vi "ModeDrivebase.vi"(0 "Master State In":T1(ring)) -> (1 "Drive Mode Change":bool, 2 "Drive Mode":enum16{"Driver Control", "Lock Heading"}(ring), 3 "Locked Heading (deg)":dbl)   [LabVIEW 2020]
doc: "This VI manages the robot drivebase mode. The default mode is driver control in which the swerve drive accepts all drive inputs and seemlessly combines them with autonomous heading corrections. Two auto targeting modes are also implimented."
uses:
  <vilib>/Rock Robotics/WPI/DriverStation/WPI_DriverStationAllianceInfo.ctl
  74109b1a-375b-4193-a712-f625c004fbb2.vi
  654a9305-fb99-4107-9368-618fc6918f82.vi
  fc0623c4-a7ba-4d2c-8dc2-a77ada9ce4c8.vi
  434b5739-c420-4379-a725-382a96265523.vi
  GlobalDriverStationCommands.vi
  GlobalPoseAndTargeting.vi
  GlobalDriverStationData.vi
  GlobalDrivebase.vi
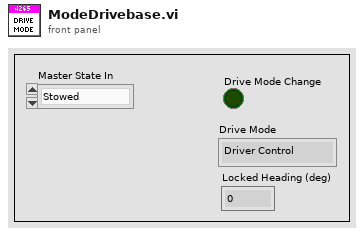
[diagram p1: front panel]
types:
  T1 = enum16{"Stowed", "Balancing", "Scoring", "Hoppering", "Ground", "Shelf"}
  T2 = enum16{"AutoTargeting", "Driver Control", "Lock Heading"}
  T3 = typedef "WPI_DriverStationAllianceInfo.ctl" = enum16{"Red", "Blue", "Invalid"}
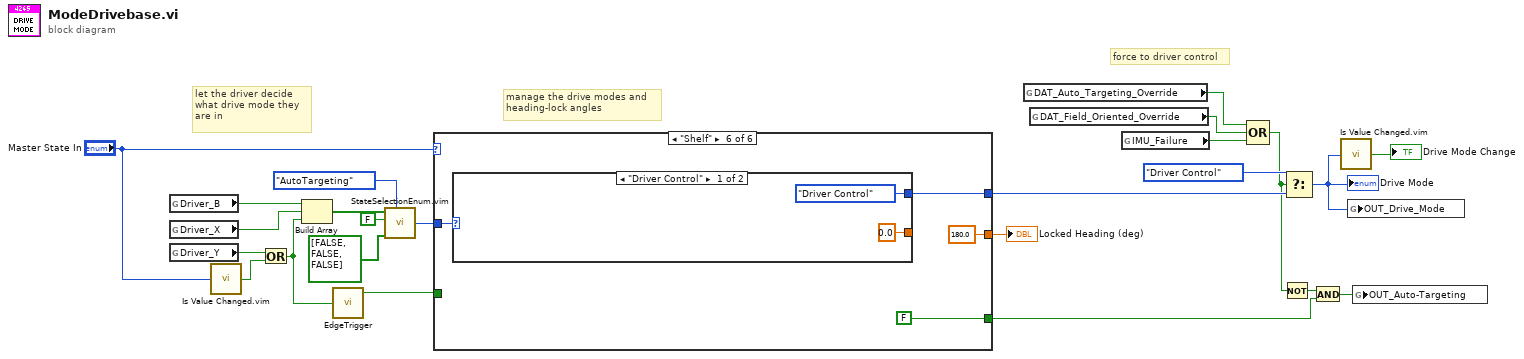
[diagram p0: block diagram]
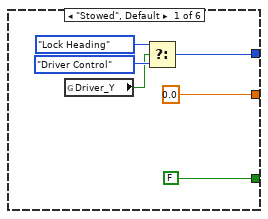
[diagram p2: hidden frame]
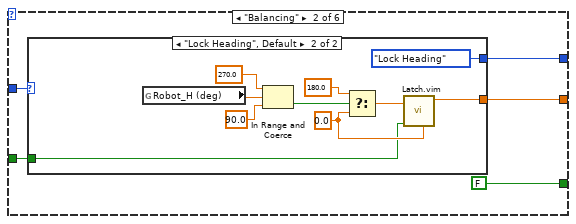
[diagram p3: hidden frame]
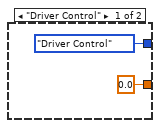
[diagram p4: hidden frame]
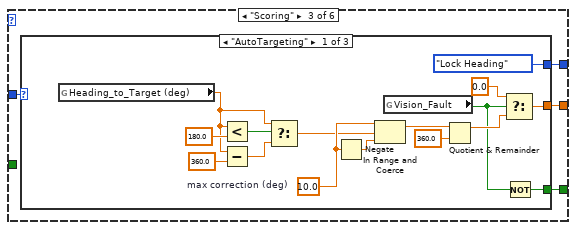
[diagram p5: hidden frame]
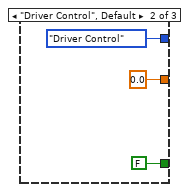
[diagram p6: hidden frame]
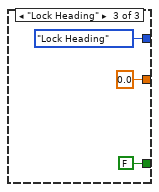
[diagram p7: hidden frame]
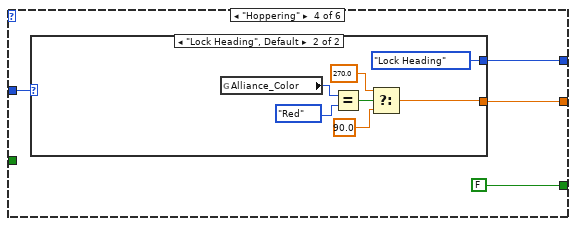
[diagram p8: hidden frame]
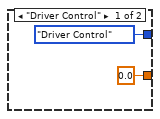
[diagram p9: hidden frame]
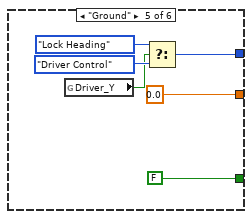
[diagram p10: hidden frame]
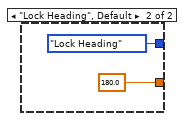
[diagram p11: hidden frame]
diagram:
  # "manage the drive modes and\nheading-lock angles"
  # "let the driver decide\nwhat drive mode they\nare in"
  # "force to driver control"
  n1 = global read "GlobalDriverStationCommands.vi" "Driver_B"() -> (w7:bool)
  n2 = global read "GlobalDriverStationCommands.vi" "Driver_X"() -> (w24:bool)
  n3 = global read "GlobalDriverStationCommands.vi" "Driver_Y"() -> (w23:bool)
  n4 = call "Is Value Changed.vim"("value"="Master State In") -> ("changed or first call?"=w13:bool)
  n5 = Or(x=w23, y=w13) -> (x .or. y?=w6:bool)
  n6 = Build Array(w7, w24, w6) -> (w22:bool[])
  n7 = call "EdgeTrigger.vi"("Input Signal"=w6) -> ("Rising Edge Trigger"=w5:bool)  [unwired: 2 out]
  n8 = call "StateSelectionEnum.vim"("Enum Def"=T2."AutoTargeting" ("Drive Mode"), "Disallowed States"=bool[] [FALSE, FALSE, FALSE], "Enable Edge Trigger"=FALSE, "State Triggers"=w22) -> ("Selected State"=w16:T2)  [unwired: 1 in, 1 out]
  n9 = case shown="\"Shelf\"" "Master State In" {
    tunnel: w16 -> [_ w33 w51 w75 _ w95]
    tunnel: [w27 w35 w50 w77 w87 w96] -> w15
    tunnel: [0.0 w34 w49 w76 0.0 180.0 ("f")] -> w14
    tunnel: w5 -> [_ w32 _ _ _ _]
    tunnel: [FALSE FALSE w48 FALSE FALSE FALSE] -> w2
    frame "Stowed", Default {
      n10 = global read "GlobalDriverStationCommands.vi" "Driver_Y"() -> (w25:bool)
      n11 = Select(t=enum16{"Driver Control", "Lock Heading"}."Lock Heading" ("Drive Mode"), s=w25, f=enum16{"Driver Control", "Lock Heading"}."Driver Control" ("Drive Mode")) -> (s? t:f=w27:enum16{"Driver Control", "Lock Heading"})
    }
    frame "Balancing" {
      n12 = case shown="\"Lock Heading\", Default" w33 {
        tunnel: [enum16{"Driver Control", "Lock Heading"}."Driver Control" ("Drive Mode") enum16{"Driver Control", "Lock Heading"}."Lock Heading" ("Drive Mode")] -> w35
        tunnel: [0.0 w40] -> w34
        tunnel: w32 -> [_ w38]
        frame "Driver Control" {
        }
        frame "Lock Heading", Default {
          w39 = 0.0 ("f")
          n13 = global read "GlobalPoseAndTargeting.vi" "Robot_H (deg)"() -> (w45:dbl)
          n14 = In Range and Coerce(upper limit=270.0, x=w45, lower limit=90.0) -> (In Range?=w46:bool)  [unwired: 1 out]
          n15 = Select(t=180.0, s=w46, f=w39) -> (s? t:f=w41:dbl)
          n16 = call "Latch.vim"("Default Value"=w39, "Latch Signal"=w38, "Latch Value"=w41) -> ("Latched"=w40:dbl)  [unwired: 8 in]
        }
      }
    }
    frame "Scoring" {
      n17 = case shown="\"AutoTargeting\"" w51 {
        tunnel: [enum16{"Driver Control", "Lock Heading"}."Lock Heading" ("Drive Mode") enum16{"Driver Control", "Lock Heading"}."Driver Control" ("Drive Mode") enum16{"Driver Control", "Lock Heading"}."Lock Heading" ("Drive Mode")] -> w50
        tunnel: [w56 0.0 0.0] -> w49
        tunnel: [w53 FALSE FALSE] -> w48
        frame "AutoTargeting" {
          w65 = 10.0  # max correction (deg)
          n18 = global read "GlobalPoseAndTargeting.vi" "Heading_to_Target (deg)"() -> (w59:dbl)
          n19 = Less?(x=w59, y=180.0) -> (x < y?=w62:bool)
          n20 = Subtract(x=w59, y=360.0) -> (x-y=w58:dbl)
          n21 = Select(t=w59, s=w62, f=w58) -> (s? t:f=w57:dbl)
          n22 = Negate(x=w65) -> (-x=w64:dbl)
          n23 = In Range and Coerce(upper limit=w65, x=w57, lower limit=w64) -> (coerced(x)=w67:dbl)  [unwired: 1 out]
          n24 = global read "GlobalPoseAndTargeting.vi" "Vision_Fault"() -> (w52:bool)
          n25 = Quotient & Remainder(x=w67, y=360.0) -> (x-y*floor(x/y)=w55:dbl)  [unwired: 1 out]
          n26 = Select(t=0.0, s=w52, f=w55) -> (s? t:f=w56:dbl)
          n27 = Not(x=w52) -> (.not. x?=w53:bool)
        }
        frame "Driver Control", Default {
        }
        frame "Lock Heading" {
        }
      }
    }
    frame "Hoppering" {
      n28 = case shown="\"Lock Heading\", Default" w75 {
        tunnel: [enum16{"Driver Control", "Lock Heading"}."Driver Control" ("Drive Mode") enum16{"Driver Control", "Lock Heading"}."Lock Heading" ("Drive Mode")] -> w77
        tunnel: [0.0 w80] -> w76
        frame "Driver Control" {
        }
        frame "Lock Heading", Default {
          n29 = global read "GlobalDriverStationData.vi" "Alliance_Color"() -> (w85:T3)
          n30 = Equal?(x=w85, y=WPI_DriverStationAllianceInfo."Red") -> (x = y?=w83:bool)
          n31 = Select(t=270.0, s=w83, f=90.0) -> (s? t:f=w80:dbl)
        }
      }
    }
    frame "Ground" {
      n32 = global read "GlobalDriverStationCommands.vi" "Driver_Y"() -> (w88:bool)
      n33 = Select(t=enum16{"Driver Control", "Lock Heading"}."Lock Heading" ("Drive Mode"), s=w88, f=enum16{"Driver Control", "Lock Heading"}."Driver Control" ("Drive Mode")) -> (s? t:f=w87:enum16{"Driver Control", "Lock Heading"})
    }
    frame "Shelf" {
      n34 = case shown="\"Driver Control\"" w95 {
        tunnel: [enum16{"Driver Control", "Lock Heading"}."Driver Control" ("Drive Mode") enum16{"Driver Control", "Lock Heading"}."Lock Heading" ("Drive Mode")] -> w96
        tunnel: [0.0 180.0] -> _
        frame "Driver Control" {
        }
        frame "Lock Heading", Default {
        }
      }
    }
  }
  "Locked Heading (deg)" <- w14
  n35 = global read "GlobalDrivebase.vi" "DAT_Auto_Targeting_Override"() -> (w8:bool)
  n36 = global read "GlobalDrivebase.vi" "DAT_Field_Oriented_Override"() -> (w17:bool)
  n37 = global read "GlobalPoseAndTargeting.vi" "IMU_Failure"() -> (w18:bool)
  n38 = Compound Arithmetic op=OR(w8, w17, w18) -> (w3:bool)
  n39 = Not(x=w3) -> (.not. x?=w4:bool)
  n40 = Select(t=enum16{"Driver Control", "Lock Heading"}."Driver Control" ("Drive Mode"), s=w3, f=w15) -> (s? t:f=w10:enum16{"Driver Control", "Lock Heading"})
  "Drive Mode" <- w10
  n41 = And(x=w4, y=w2) -> (x .and. y?=w1:bool)
  n42 = call "Is Value Changed.vim"("value"=w10) -> ("changed or first call?"=→"Drive Mode Change":bool)
  n43 = global write "GlobalDrivebase.vi" "OUT_Drive_Mode"(w10) -> ()
  n44 = global write "GlobalDrivebase.vi" "OUT_Auto-Targeting"(w1) -> ()
